vi "CellClick Event Callback.vi"(4 "User Parameter":variant, 5 "Event Data":cluster{"sender":refnum<k24>, "e":refnum<k24>}, 6 "Control Ref":refnum<k24>, 7 "Event Common Data":T1) -> ()   [LabVIEW 2014]
uses:
  System.Windows.Forms
  <vilib>/Platform/browser.llb/Open URL in Default Browser (string).vi
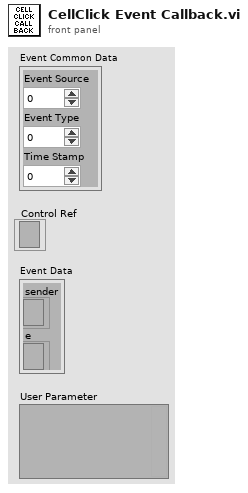
[diagram p1: front panel]
types:
  T1 = cluster{"Event Source":i32, "Event Type":u32, "Time Stamp":u32}
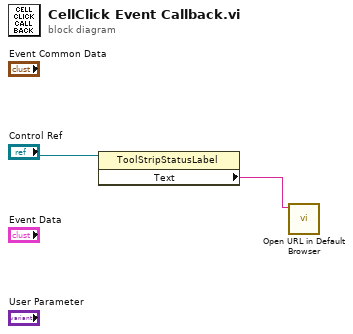
[diagram p0: block diagram]
diagram:
  n1 = property class="ToolStripStatusLabel"(reference="Control Ref") -> ("Text"=w1:string)  [unwired: 1 in, 2 out]
  n2 = call-poly <vilib>:"Open URL in Default Browser.vi"("URL"=w1) -> ()  [unwired: 5 in, 2 out]
